vi "CheckifMoveComplete.vi"(8 "error in (no error)":errorcluster) -> (0 "error out 2":errorcluster, 2 "x = y? 2":bool)   [LabVIEW 2018]
uses:
  <vilib>/regexp/Match Regular Expression.xnode
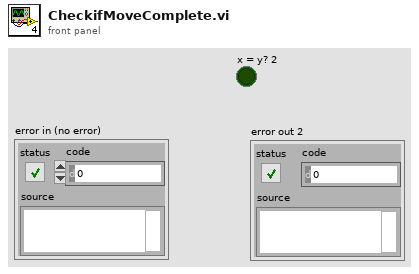
[diagram p1: front panel]
types:
  T1 = enum16{"Standard", "Buffered", "CRLF", "Immediate"}
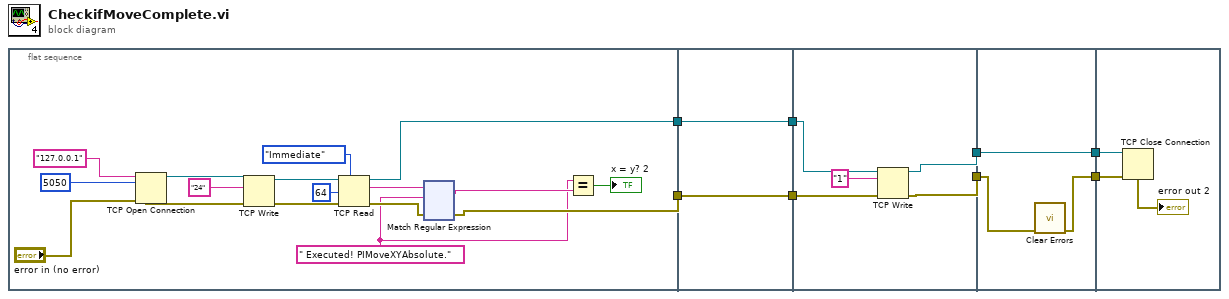
[diagram p0: block diagram]
diagram:
  n1 = flat-sequence {
    tunnel: [w15] -> w8
    tunnel: [w12] -> w1
    tunnel: w8 -> [w141]
    tunnel: [w141] -> w3
    tunnel: [w140] -> w2
    tunnel: w1 -> [w140]
    tunnel: [w144] -> w7
    tunnel: [w143] -> w6
    tunnel: w3 -> [w146]
    tunnel: w2 -> [w142]
    tunnel: [w147] -> w5
    tunnel: w7 -> [w148]
    tunnel: [w149] -> w4
    tunnel: w6 -> [w149]
    tunnel: w5 -> [w151]
    tunnel: w4 -> [w150]
    frame #0 {
      w9 = " Executed! PIMoveXYAbsolute." ("y")
      n2 = TCP Open Connection(address="127.0.0.1", remote port or service name=u16 5050, error in (no error)="error in (no error)") -> (connection ID=w18:refnum<k5>, error out=w17:errorcluster)  [unwired: 2 in]
      n3 = TCP Write(connection ID=w18, data in="24", error in (no error)=w17) -> (connection ID out=w23:refnum<k5>, error out=w24:errorcluster)  [unwired: 1 in, 1 out]
      n4 = TCP Read(connection ID=w23, bytes to read=64, error in (no error)=w24, 7:T1."Immediate" ("mode (standard)")) -> (connection ID out=w15:refnum<k5>, data out=w14:string, error out=w13:errorcluster)  [unwired: 1 in]
      n5 = xnode "Match Regular Expression"("input string"=w14, "regular expression"=w9, "error in"=w13) -> ("whole match"=w10:string, "error out"=w12:errorcluster)  [unwired: 3 in, 3 out]
      n6 = Equal?(x=w9, y=w10) -> (x = y?=→"x = y? 2":bool)
    }
    frame #1 {
    }
    frame #2 {
      n7 = TCP Write(connection ID=w146, data in="1", error in (no error)=w142) -> (connection ID out=w143:refnum<k5>, error out=w144:errorcluster)  [unwired: 1 in, 1 out]
    }
    frame #3 {
      n8 = call <vilib>:"Clear Errors.vi"("error in (no error)"=w148) -> ("error out"=w147:errorcluster)  [unwired: 5 in, 1 out]
    }
    frame #4 {
      n9 = TCP Close Connection(connection ID=w150, error in (no error)=w151) -> (error out=→"error out 2":errorcluster)  [unwired: 1 in, 1 out]
    }
  }
